vi "Decode Balls.vi"(5 "Time Stamp":timestamp, 8 "error in":errorcluster, 9 "array":u8[](array[numeric]), 10 "Key":i32=5) -> (0 "error out":errorcluster, 1 "array w/ subset deleted out":u8[](array[numeric]), 3 "Array":refnum<class "Ball.lvclass">[](array[class]))   [LabVIEW 2018]
uses:
  Ball_class/Ball.lvclass
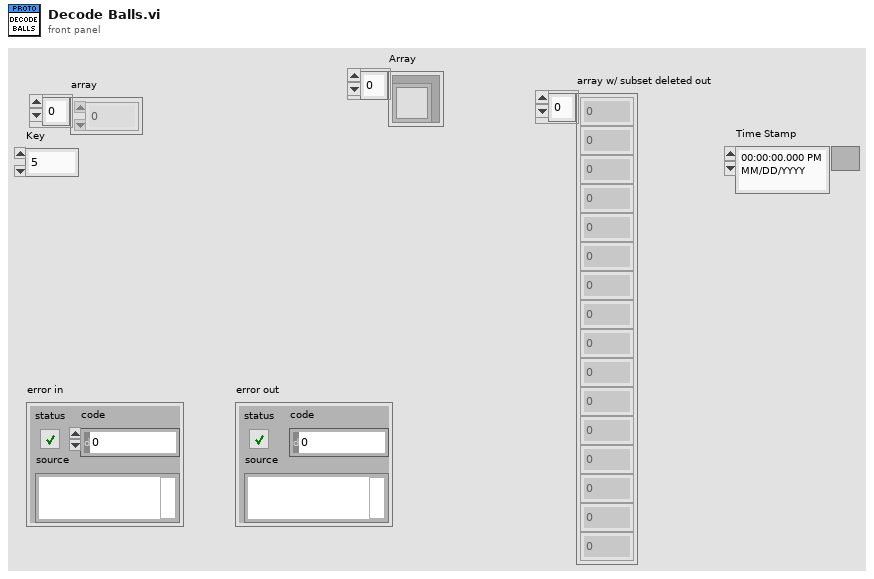
[diagram p1: front panel]
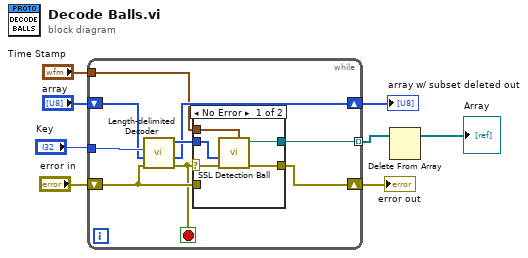
[diagram p0: block diagram]
diagram:
  n1 = while {
    shift-right: [w15] -> w6
    shift-left: "array" -> [w11]
    shift-right: [w17] -> w8
    shift-left: "error in" -> [w14]
    tunnel: "Key" -> [w12]
    tunnel: "Time Stamp" -> [w10]
    tunnel: [w9] -> w2 mode=indexing
    stop <- w13 stop-if-true
    n2 = call "Length-delimited Decoder.vi"("error in (no error)"=w14, "Array"=w11, "Key"=w12) -> ("error out"=w13:errorcluster, "array w/ subset deleted"=w15:u8[], "Length-delimited"=w16:u8[])  [unwired: 5 in, 1 out]
    n3 = case shown="No Error" w13 {
      selector: w13 -> [w21 _]
      tunnel: [w22 w23] -> w17
      tunnel: w16 -> [w20 _]
      tunnel: w14 -> [_ w23]
      tunnel: w10 -> [w19 _]
      tunnel: [w18 _] -> w9
      frame No Error {
        n4 = call "SSL Detection Ball.vi"("Time Stamp"=w19, "error in"=w21, "Array"=w20) -> ("error out"=w22:errorcluster, "Detection Ball"=w18:refnum<class "Ball.lvclass">)  [unwired: 6 in, 1 out]
      }
      frame Error {
      }
    }
  }
  "error out" <- w8
  "array w/ subset deleted out" <- w6
  n5 = Delete From Array(array=w2) -> (array with subset deleted=→"Array":refnum<class "Ball.lvclass">[])  [unwired: 2 in, 1 out]
